vi "LCC Lookup Ctrl Device By Name.vi"(7 "error in (no error)":errorcluster caption="Fehler (Eingang, kein Fehler)", 10 "Device Name":string) -> (0 "error out":errorcluster caption="Fehler (Ausgang)", 3 "Controller Device Handle":i64)   [LabVIEW 2021, in "labbCAN_Controller_API.lvlib"]
doc: "LCC_Func long LCC_CALL LCC_LookupCtrlDeviceByName(char *pName,\n dev_hdl *pCtrlDeviceHdl);"
uses:
  labbCAN_Controller_API.lvlib
  labbCAN_Controller_API.dll
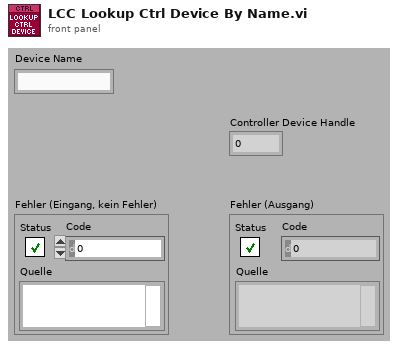
[diagram p1: front panel]
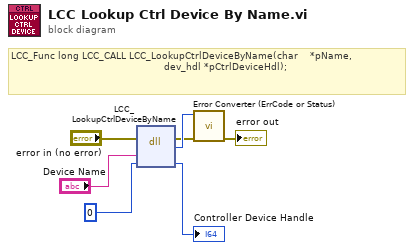
[diagram p0: block diagram]
diagram:
  # "LCC_Func long LCC_CALL LCC_LookupCtrlDeviceByName(char    *pName,\n                                                   dev_hdl *pCtrlDeviceHdl);"
  n1 = dll-call lib="C:/Users/olaja/AppData/Local/CETONI_SDK/labbCAN_Controller_API.*" fn="LCC_LookupCtrlDeviceByName"(error in="error in (no error)", "pName"="Device Name", "pCtrlDeviceHdl"=i64 0) -> (error out=w2:errorcluster, "Rückgabetyp"=w3:i32, "pCtrlDeviceHdl"=→"Controller Device Handle":i64)  [unwired: 3 in, 1 out]
  n2 = call "Error Converter (ErrCode or Status).vi"("error in (no error)"=w2, "error code"=w3) -> ("error out"=→"error out":errorcluster)  [unwired: 9 in]
